vi "Database_C_U.vi"(8 "error in (no error)":errorcluster, 9 "Basic_info":string[](array[string])=["'DUT'", "'Module'", "'operator'", "'123'"], 10 "Values":string[](array[string])=["0", "0", "0", "0", "0", "0", "0", "0", "0", "0", "0", "0", "0", "0", "0", "0", "0", "0", "0", "0", "0", "0", "0", "0"], 11 "Combo Box":string(combo)) -> (0 "error out":errorcluster, 1 "Result":bool)   [LabVIEW 2021]
panel:
  out "standard error 2":string
  out "standard error":string
  out "concatenated string":string
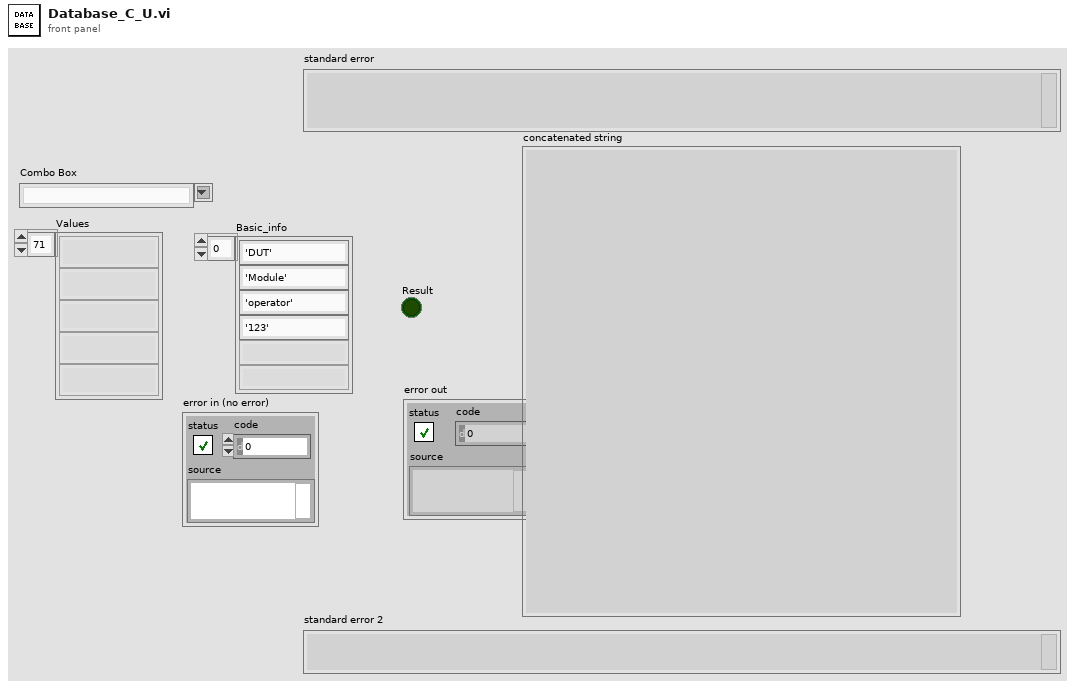
[diagram p1: front panel]
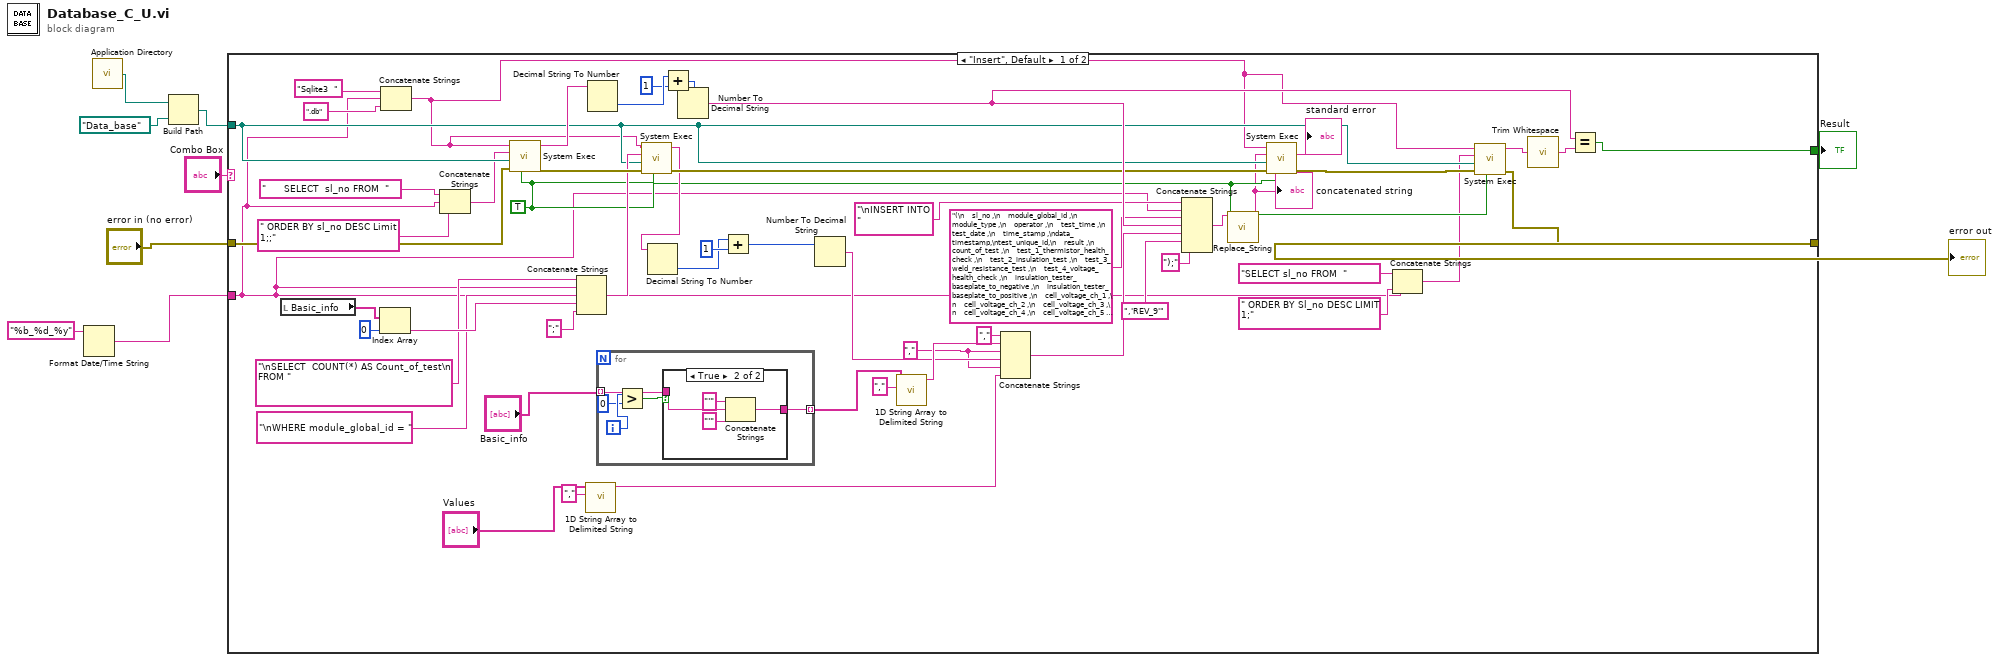
[diagram p0: block diagram]
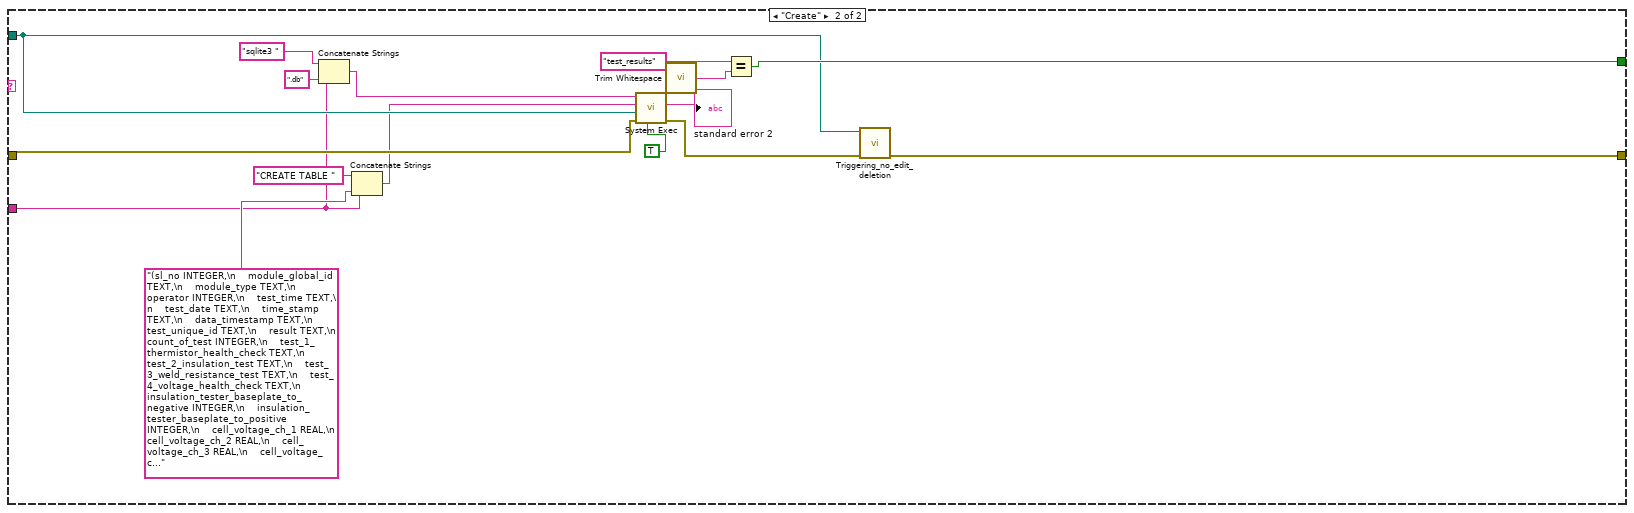
[diagram p3: hidden frame]
diagram:
  n1 = Format Date/Time String(time format string (%c)="%b_%d_%y") -> (date/time string=w3:string)  [unwired: 2 in]
  n2 = call <vilib>:"Application Directory.vi"() -> ("Application Directory"=w2:path)
  n3 = Build Path(base path=w2, name or relative path=path "Data_base" ("working directory")) -> (appended path=w1:path)
  n4 = case shown="\"Insert\", Default" "Combo Box" {
    tunnel: "error in (no error)" -> [w63 w90]
    tunnel: [w53 w85] -> w7
    tunnel: w1 -> [w31 w83]
    tunnel: [w54 w86] -> w6
    tunnel: w3 -> [w13 w75]
    frame "Insert", Default {
      w38 = "," ("string")
      w30 = TRUE ("run minimized? (F)")
      n5 = local read "Basic_info"() -> (w49:string[])
      n6 = Index Array(array=w49, index=0) -> (element=w19:string)
      n7 = Concatenate Strings("Sqlite3  " ("command line"), w13, ".db" ("string")) -> (w15:string)
      n8 = Concatenate Strings("      SELECT  sl_no FROM  " ("standard input"), w13, " ORDER BY sl_no DESC Limit 1;;" ("standard input")) -> (w28:string)
      n9 = call <vilib>:"System Exec.vi"("run minimized? (F)"=w30, "error in (no error)"=w63, "working directory"=w31, "standard input"=w28, "command line"=w15) -> ("error out"=w52:errorcluster, "standard output"=w62:string)  [unwired: 3 in, 2 out]
      n10 = Concatenate Strings("\nSELECT  COUNT(*) AS Count_of_test\n   FROM ", w13, "\nWHERE module_global_id = ", w19, ";" ("string")) -> (w33:string)
      n11 = call <vilib>:"1D String Array to Delimited String.vi"("delimiter"=",", "string array"="Values") -> ("delimited string"=w37:string)  [unwired: 9 in]
      n12 = Decimal String To Number(string=w62) -> (number=w61:i32)  [unwired: 2 in, 1 out]
      n13 = for {
        tunnel: "Basic_info" -> [w65] mode=indexing
        tunnel: [w64] -> w34 mode=indexing
        i -> [w68]
        n14 = Greater?(x=w68, y=0) -> (0:w66:bool)
        n15 = case shown="True" w66 {
          tunnel: w65 -> [w69 w71]
          tunnel: [w69 w70] -> w64
          frame False {
          }
          frame True {
            n16 = Concatenate Strings("'" ("string"), w71, "'" ("string")) -> (w70:string)
          }
        }
      }
      n17 = call <vilib>:"System Exec.vi"("run minimized? (F)"=w30, "error in (no error)"=w52, "working directory"=w31, "standard input"=w33, "command line"=w15) -> ("error out"=w51:errorcluster, "standard output"=w32:string)  [unwired: 3 in, 2 out]
      n18 = Decimal String To Number(string=w32) -> (number=w46:i32)  [unwired: 2 in, 1 out]
      n19 = Add(x=w61, y=1) -> (x+y=w59:i32)
      n20 = Number To Decimal String(number=w59) -> (decimal integer string=w55:string)  [unwired: 1 in]
      n21 = Add(x=w46, y=1) -> (x+y=w45:i32)
      n22 = Number To Decimal String(number=w45) -> (decimal integer string=w41:string)  [unwired: 1 in]
      n23 = call <vilib>:"1D String Array to Delimited String.vi"("delimiter"=",", "string array"=w34) -> ("delimited string"=w43:string)  [unwired: 9 in]
      n24 = Concatenate Strings("," ("string"), w43, w38, w41, w38, w37) -> (w42:string)
      n25 = Concatenate Strings("\nINSERT INTO " ("string"), w13, "(\n    sl_no ,\n    module_global_id ,\n    module_type ,\n    operator ,\n    test_time ,\n    test_date ,\n    time_stamp ,\ndata_timestamp,\ntest_unique_id,\n    result ,\n    count_of_test ,\n    test_1_thermistor_health_check ,\n    test_2_insulation_test ,\n    test_3_weld_resistance_test ,\n    test_4_voltage_health_check ,\n    insulation_tester_baseplate_to_negative ,\n    insulation_tester_baseplate_to_positive ,\n    cell_voltage_ch_1 ,\n    cell_voltage_ch_2 ,\n    cell_voltage_ch_3 ,\n    cell_voltage_ch_4 ,\n    cell_voltage_ch_5 ,\n    cell_voltage_ch_6 ,\n    cell_voltage_ch_7 ,\n    cell_voltage_ch_8 ,\n    max_voltage ,\n    min_voltage ,\n    s8_voltage ,\n    s8_voltage_imbalance ,\n    thermistor_ch_1 ,\n    thermistor_ch_2 ,\n    thermistor_ch_3 ,\n    ambient_temperature ,\n    max_temperature ,\n    min_temperature ,\n    s8_temperature_imbalance ,\n    ambient_temperature_imbalance ,\n    weld_resistance_ch_1 ,\n    weld_resistance_ch_2 ,\n    weld_resistance_ch_3 ,\n    weld_resistance_ch_4 ,\n    weld_resistance_ch_5 ,\n    weld_resistance_ch_6 ,\n    weld_resistance_ch_7 ,\n    weld_resistance_ch_8 ,\n    weld_resistance_ch_9 ,\n    weld_voltage_1_uv ,\n    weld_voltage_2_uv ,\n    weld_voltage_3_uv ,\n    weld_voltage_4_uv ,\n    weld_voltage_5_uv ,\n    weld_voltage_6_uv ,\n    weld_voltage_7_uv ,\n    weld_voltage_8_uv ,\n    weld_voltage_9_uv ,\n    load_current ,\n    cell_1_end_busbar_min ,\n    cell_1_end_busbar_max ,\n    cell_1_cell_2_min ,\n    cell_1_cell_2_max ,\n    cell_2_cell_3_min ,\n    cell_2_cell_3_max ,\n    cell_3_cell_4_min ,\n    cell_3_cell_4_max ,\n    cell_4_cell_5_min ,\n    cell_4_cell_5_max ,\n    cell_5_cell_6_min ,\n    cell_5_cell_6_max ,\n    cell_6_cell_7_min ,\n    cell_6_cell_7_max ,\n    cell_7_cell_8_min ,\n    cell_7_cell_8_max ,\n    cell_8_end_busbar_min ,\n    cell_8_end_busbar_max ,\n\n    insulation_test_min ,\n    insulation_test_max ,\n    voltage_health_test_min ,\n    voltage_health_test_max ,\n    temperature_imbalance_min ,\n    temperature_imbalance_max ,\n    temperature_ambient_min ,\n    temperature_ambient_max ,\n    cell_voltage_min ,\n    cell_voltage_max ,\nsensor_type,\nvariant_type,\n    limits_revision ,\n    application_revision  ) \nVALUES(" ("standard input"), w55, w42, ",'REV_9'" ("string"), ");" ("string")) -> (w11:string)
      n26 = call "Replace_String.vi"("input string"=w11) -> ("result string"=w10:string)  [unwired: 10 in]
      "concatenated string" <- w10
      n27 = call <vilib>:"System Exec.vi"("run minimized? (F)"=w30, "error in (no error)"=w51, "working directory"=w31, "standard input"=w10, "command line"=w15) -> ("error out"=w58:errorcluster, "standard error"=→"standard error":string)  [unwired: 3 in, 2 out]
      n28 = Concatenate Strings("SELECT sl_no FROM  " ("standard input"), w13, " ORDER BY Sl_no DESC LIMIT 1;" ("standard input")) -> (w20:string)
      n29 = call <vilib>:"System Exec.vi"("run minimized? (F)"=w30, "error in (no error)"=w58, "working directory"=w31, "standard input"=w20, "command line"=w15) -> ("error out"=w53:errorcluster, "standard output"=w57:string)  [unwired: 3 in, 2 out]
      n30 = call <vilib>:"Trim Whitespace.vi"("string"=w57) -> ("trimmed string"=w56:string)  [unwired: 1 in]
      n31 = Equal?(x=w55, y=w56) -> (x = y?=w54:bool)
    }
    frame "Create" {
      n32 = Concatenate Strings("sqlite3 ", w75, ".db" ("string")) -> (w77:string)
      n33 = Concatenate Strings("CREATE TABLE " ("string"), w75, "(sl_no INTEGER,\n    module_global_id TEXT,\n    module_type TEXT,\n    operator INTEGER,\n    test_time TEXT,\n    test_date TEXT,\n    time_stamp TEXT,\n    data_timestamp TEXT,\n    test_unique_id TEXT,\n    result TEXT,\n    count_of_test INTEGER,\n    test_1_thermistor_health_check TEXT,\n    test_2_insulation_test TEXT,\n    test_3_weld_resistance_test TEXT,\n    test_4_voltage_health_check TEXT,\n    insulation_tester_baseplate_to_negative INTEGER,\n    insulation_tester_baseplate_to_positive INTEGER,\n    cell_voltage_ch_1 REAL,\n    cell_voltage_ch_2 REAL,\n    cell_voltage_ch_3 REAL,\n    cell_voltage_ch_4 REAL,\n    cell_voltage_ch_5 REAL,\n    cell_voltage_ch_6 REAL,\n    cell_voltage_ch_7 REAL,\n    cell_voltage_ch_8 REAL,\n    max_voltage REAL,\n    min_voltage REAL,\n    s8_voltage REAL,\n    s8_voltage_imbalance REAL,\n    thermistor_ch_1 REAL,\n    thermistor_ch_2 REAL,\n    thermistor_ch_3 REAL,\n    ambient_temperature REAL,\n    max_temperature REAL,\n    min_temperature REAL,\n    s8_temperature_imbalance REAL,\n    ambient_temperature_imbalance REAL,\n    weld_resistance_ch_1 REAL,\n    weld_resistance_ch_2 REAL,\n    weld_resistance_ch_3 REAL,\n    weld_resistance_ch_4 REAL,\n    weld_resistance_ch_5 REAL,\n    weld_resistance_ch_6 REAL,\n    weld_resistance_ch_7 REAL,\n    weld_resistance_ch_8 REAL,\n    weld_resistance_ch_9 REAL,\n    weld_voltage_1_uv REAL,\n    weld_voltage_2_uv REAL,\n    weld_voltage_3_uv REAL,\n    weld_voltage_4_uv REAL,\n    weld_voltage_5_uv REAL,\n    weld_voltage_6_uv REAL,\n    weld_voltage_7_uv REAL,\n    weld_voltage_8_uv REAL,\n    weld_voltage_9_uv REAL,\n    load_current REAL,\n    cell_1_end_busbar_min REAL,\n    cell_1_end_busbar_max REAL,\n    cell_1_cell_2_min REAL,\n    cell_1_cell_2_max REAL,\n    cell_2_cell_3_min REAL,\n    cell_2_cell_3_max REAL,\n    cell_3_cell_4_min REAL,\n    cell_3_cell_4_max REAL,\n    cell_4_cell_5_min REAL,\n    cell_4_cell_5_max REAL,\n    cell_5_cell_6_min REAL,\n    cell_5_cell_6_max REAL,\n    cell_6_cell_7_min REAL,\n    cell_6_cell_7_max REAL,\n    cell_7_cell_8_min REAL,\n    cell_7_cell_8_max REAL,\n    cell_8_end_busbar_min REAL,\n    cell_8_end_busbar_max REAL,\n    insulation_test_min REAL,\n    insulation_test_max REAL,\n    voltage_health_test_min REAL,\n    voltage_health_test_max REAL,\n    temperature_imbalance_min REAL,\n    temperature_imbalance_max REAL,\n    temperature_ambient_min REAL,\n    temperature_ambient_max REAL,\n    cell_voltage_min REAL,\n    cell_voltage_max REAL,\nsensor_type TEXT,\nvariant_type TEXT,\n    limits_revision REAL,\n    application_revision TEXT);" ("standard input")) -> (w79:string)
      n34 = call <vilib>:"System Exec.vi"("run minimized? (F)"=TRUE, "error in (no error)"=w90, "working directory"=w83, "standard input"=w79, "command line"=w77) -> ("error out"=w84:errorcluster, "standard error"=→"standard error 2":string, "standard output"=w89:string)  [unwired: 3 in, 1 out]
      n35 = call <vilib>:"Trim Whitespace.vi"("string"=w89) -> ("trimmed string"=w87:string)  [unwired: 1 in]
      n36 = Equal?(x="test_results", y=w87) -> (x = y?=w86:bool)
      n37 = call "Triggering_no_edit_deletion.vi"("error in (no error)"=w84, "working directory"=w83) -> ("error out"=w85:errorcluster)  [unwired: 9 in]
    }
  }
  "error out" <- w7
  "Result" <- w6
